vi "Read configuration.vi"(8 "error in":errorcluster, 11 "cfg cRIO root in":refnum<class "cfg cRIO root.lvclass">) -> (0 "error out":errorcluster, 2 "configuration":refnum<class "NISE_CEF_serializable configuration.lvclass">, 3 "cfg cRIO root out":refnum<class "cfg cRIO root.lvclass">)   [LabVIEW 2013, in "cfg cRIO root.lvclass"]
uses:
  cfg cRIO root.lvclass
  CEF_TreeControl/serializable configuration/NISE_CEF_serializable configuration.lvclass
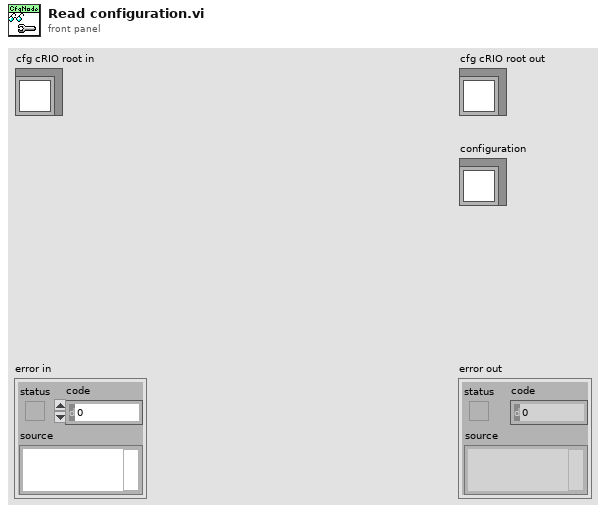
[diagram p1: front panel]
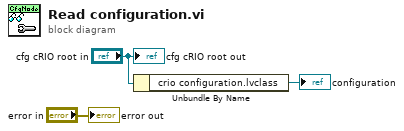
[diagram p0: block diagram]
diagram:
  n1 = Unbundle By Name("cfg cRIO root in") -> ("crio configuration.lvclass"=→"configuration":refnum<class "crio configuration.lvclass">)
  "error out" <- "error in"
  "cfg cRIO root out" <- "cfg cRIO root in"
